vi "IMUPeriodic.vi"(8 "error in":errorcluster) -> (0 "error out":errorcluster)   [LabVIEW 2014]
uses:
  NavX/roborio/labview/navX-MXP Library/COMMON/TypeDefs/Data TypeDefs/navX Vector Data.ctl
  NavX/roborio/labview/navX-MXP Library/navX-MXP IMU.lvlib
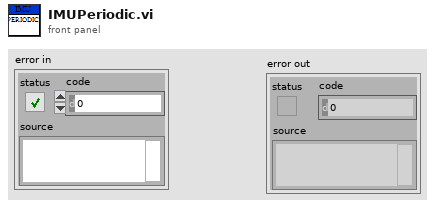
[diagram p1: front panel]
types:
  T1 = typedef "navX-MXP IMU.lvlib/navX Vector Data.ctl" = cluster{"X":dbl, "Y":dbl, "Z":dbl}
  T2 = typedef "navX-MXP IMU.lvlib/navX Device TypeDef.ctl" = cluster{"navX Interface Protocol":T3, "navX Interface Protocol TypeDefs":cluster{"SPIDevRef":T4, "I2CDevRef":T7}, "navX System Information":cluster{"Board Information":T9, "Status":T10, "Offsets":T14}, "navX Common Information":cluster{"Update Rate (4Hz-60Hz)":T15, "refnum name":string, "error":errorcluster}}
  T3 = typedef "navX-MXP IMU.lvlib/navX Interface Protocol.ctl" = enum16{"SPI", "I2C"}
  T4 = typedef "WPI_SPIDevRef.ctl" = cluster{"DevStatus":errorcluster, "Handle":i32, "Controller":T5, "SPI Bus":T6}
  T5 = typedef "FPGA_TypedefDigitalModule.ctl" = enum16{"Controller 1"}
  T6 = typedef "spi_bus.ctl" = enum16{"SPI On-Board, CS0", "SPI On-Board, CS1", "SPI On-Board, CS2", "SPI On-Board, CS3", "SPI MXP", "Invalid"}
  T7 = typedef "WPI_I2CDevRef.ctl" = cluster{"DevStatus":errorcluster, "Controller":T5, "Device Address":u8, "Handle":i32, "I2C Bus":T8}
  T8 = typedef "i2c_bus.ctl" = enum16{"I2C On-Board", "I2C MXP", "Invalid"}
  T9 = typedef "navX-MXP IMU.lvlib/navX Board Information.ctl" = cluster{"WhoAmI (50 | 0x32)":u8, "Board Revision":u8, "Firmware Major Version":u8, "Firmware Minor Version":u8}
  T10 = typedef "navX-MXP IMU.lvlib/navX Status Data.ctl" = cluster{"Update Rate Hz":u8, "Accelerometer Full-Scale Range":u8, "Gyro Full-Scale Range":u16, "NAVX_OP_STATUS":T11, "NAVX_CAL_STATUS":T12, "NAVX_SELFTEST_STATUS":u8, "NAVX_SENSOR_STATUS":T13}
  T11 = typedef "navX-MXP IMU.lvlib/navX NAVX_OP_STATUS.ctl" = u8
  T12 = typedef "navX-MXP IMU.lvlib/navX NAVX_CAL_STATUS.ctl" = u8
  T13 = typedef "navX-MXP IMU.lvlib/navX NAVX_SENSOR_STATUS.ctl" = cluster{"MOVING":bool, "YAW_STABLE":bool, "MAG_DISTURBANCE":bool, "ALTITUDE_VALID":bool, "SEALEVEL_PRESS_SET":bool, "FUSED_HEADING_VALID":bool}
  T14 = typedef "navX-MXP IMU.lvlib/navX Offsets Data.ctl" = cluster{"Yaw":dbl, "Quat W":dbl, "Quat X":dbl, "Quat Y":dbl, "Quat Z":dbl}
  T15 = typedef "navX-MXP IMU.lvlib/navX Update Rate.ctl" = u8
  T16 = cluster{"P_Acc":T1, "P_Vel":T1, "P_Pos":T1, "T":i32, "navX Device TypeDef":T2}
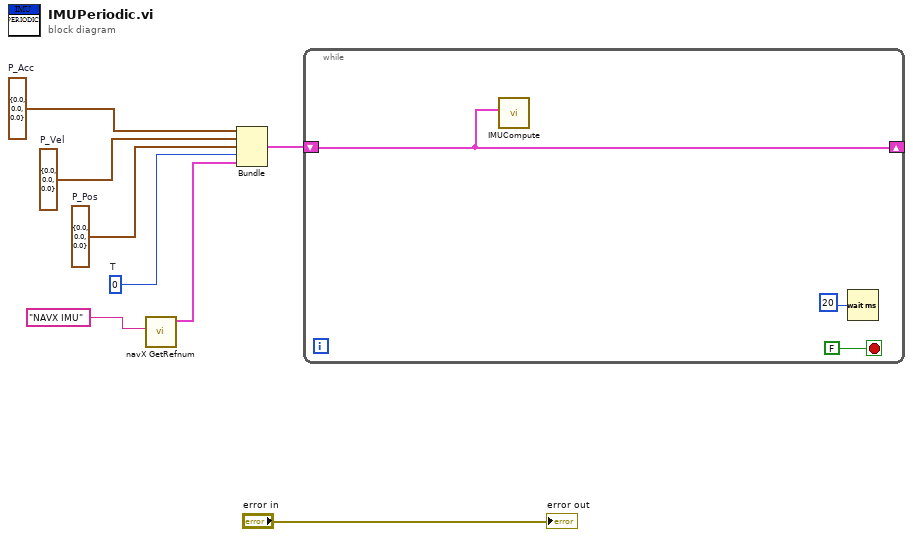
[diagram p0: block diagram]
diagram:
  w4 = 0  # T
  w5 = T1 {"X"=0.0, "Y"=0.0, "Z"=0.0}  # P_Pos
  w6 = T1 {"X"=0.0, "Y"=0.0, "Z"=0.0}  # P_Vel
  w7 = T1 {"X"=0.0, "Y"=0.0, "Z"=0.0}  # P_Acc
  n1 = call "navX GetRefnum.vi"("refnum name"="NAVX IMU") -> ("navX Device TypeDef"=w3:T2)  [unwired: 9 in, 1 out]
  n2 = Bundle("P_Acc"=w7, "P_Vel"=w6, "P_Pos"=w5, "T"=w4, "navX Device TypeDef"=w3) -> (w2:T16)  [unwired: 1 in]
  n3 = while {
    shift-right: [w9] -> _
    shift-left: w2 -> [w9]
    stop <- FALSE stop-if-true
    n4 = call "IMUCompute.vi"("Cluster"=w9) -> ()  [unwired: 11 in]
    n5 = Wait (ms)(milliseconds to wait=20) -> ()  [unwired: 1 out]
  }
  "error out" <- "error in"
